vi "PH_gentec_Powermeter.destructor.vi"(0 "i ref in":refnum<vi>, 5 "error in(no error)":errorcluster) -> (19 "error out":errorcluster)   [LabVIEW 2014, in "PH_gentec_Powermeter.lvlib"]
doc: "This is the destructor of a class.\n\nLicense Agreement for this software:\n\nCopyright (C)\nGesellschaft für Schwerionenforschung, GSI\nPlanckstr. 1\n64291 Darmstadt\nGermany\n\nContact: D.Beck@gsi.de \n\nThis program is free software; you can redistribute it and/or modify it under the terms of the \nGNU General Public License as published by the Free Software Foundation; either version 2 of \nthe license, or (at your option) any later version.\n\nThis program is distributed in the hope that it will be useful, but WITHOUT ANY WARRANTY; \nwithout even the implied warranty of MERCHANTABILITY or FITNESS FOR A PARTICULAR PURPOSE. See the GNU General License for more details (http://www.gnu.org).\n\nGesellschaft für Schwerionenforschung, GSI\nPlanckstr. 1, 64291 Darmstadt, Germany\nFor all questions and ideas contact: M.Richter@gsi.de, H.Brand@gsi.de or D.Beck@gsi.de.\nLast update: 16-JUN-2004"
uses:
  PH_gentec_Powermeter.lvlib
  PH_Powermeter_BaseClass/PH_Powermeter_BaseClass.State.ctl
  PH_Powermeter_BaseClass/PH_Powermeter_BaseClass.lvlib
  non_GPL/instr.lib/gentec-SOLO-PE/gentec-SOLO-PE - Driver.lvlib
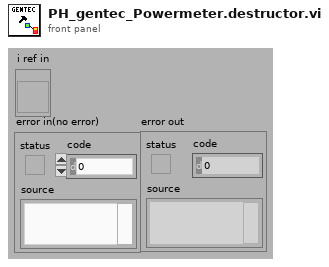
[diagram p1: front panel]
types:
  T1 = typedef "PH_Powermeter_BaseClass.lvlib/PH_Powermeter_BaseClass.State.ctl" = enum32{"off", "operating", "opened", "checked", "connected", "Sets to change", "running"}
  T2 = typedef "PH_Powermeter_BaseClass.lvlib/PH_Powermeter_BaseClass.i attribute.ctl" = cluster{"GUI References":T3, "Connection":T4, "Head Attributes":T5, "VISA resource":refnum<visa-resource-name>, "Energy":T6, "Service ID Energy":i32, "Wanted Settings":T7, "Current Settings":T7}
  T3 = typedef "PH_Powermeter_BaseClass.lvlib/PH_Powermeter_BaseClass.GUI Refs.ctl" = cluster{"Head Attributes":refnum<vi>, "Energy":refnum<vi>, "Connection":refnum<vi>, "VISA Resource":refnum<vi>, "Energy evolution":refnum<vi>, "Scaling Factor":refnum<vi>, "Range":refnum<vi>, "Wavelength":refnum<vi>, "Trigger Level":refnum<vi>, "Wanted Settings":refnum<vi>, "Current Settings":refnum<vi>}
  T4 = typedef "PH_Powermeter_BaseClass.lvlib/PH_Powermeter_BaseClass.Connection.ctl" = cluster{"failed checks":i8, "Timeout":bool, "Data read":string, "Failure":bool, "Error":bool, "State":T1}
  T5 = typedef "PH_Powermeter_BaseClass.lvlib/PH_Powermeter_BaseClass.Head Attributes.ctl" = cluster{"Instrument Type":string, "Head Version":string, "Head Name":string, "Serial Number":string, "Firmware":string, "Sensor Type":string, "MinimumRange":u32, "Maximum Range":u32, "Min Wavelength":i32, "Max Wavelength":i32}
  T6 = typedef "PH_Powermeter_BaseClass.lvlib/PH_Powermeter_BaseClass.Energy.ctl" = cluster{"current Value":dbl, "unscaled":dbl, "Scaling Factor":dbl}
  T7 = typedef "PH_Powermeter_BaseClass.lvlib/PH_gentec_BaseClass.Head Settings.ctl" = cluster{"Trigger Level":dbl, "Wavelength":u32, "Range":u32}
  T8 = enum16{"SetAttribute", "GetAttribute", "CreateAttribute", "DestroyAttribute", "DestroyAllAtributes"}
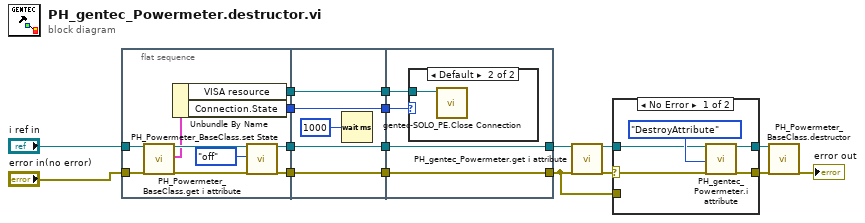
[diagram p0: block diagram]
diagram:
  n1 = flat-sequence {
    tunnel: "error in(no error)" -> [w24]
    tunnel: "i ref in" -> [w23]
    tunnel: [w26] -> w12
    tunnel: [w27] -> w11
    tunnel: [w19] -> w10
    tunnel: [w18] -> w9
    tunnel: w12 -> [w32]
    tunnel: w11 -> [w31]
    tunnel: [w32] -> w8
    tunnel: [w31] -> w7
    tunnel: w10 -> [w29]
    tunnel: [w29] -> w6
    tunnel: [w28] -> w5
    tunnel: w9 -> [w28]
    tunnel: [w34] -> w3
    tunnel: [w33] -> w2
    tunnel: w8 -> [w33]
    tunnel: w7 -> [w34]
    tunnel: w6 -> [w36]
    tunnel: w5 -> [w35]
    frame #0 {
      n2 = call "PH_Powermeter_BaseClass.get i attribute.vi"("i ref in"=w23, "error in (no error)"=w24) -> ("i ref out"=w21:refnum<vi>, "i attribute"=w20:T2, "error out"=w22:errorcluster)  [unwired: 15 in]
      n3 = Unbundle By Name(w20) -> ("VISA resource"=w19:refnum<visa-resource-name>, "Connection.State"=w18:T1)
      n4 = call "PH_Powermeter_BaseClass.set State.vi"("VI in"=w21, "State"=PH_Powermeter_BaseClass.State."off", "error in (no error)"=w22) -> ("VI out"=w27:refnum<vi>, "error out"=w26:errorcluster)  [unwired: 15 in]
    }
    frame #1 {
      n5 = Wait (ms)(milliseconds to wait=u32 1000) -> ()  [unwired: 1 out]
    }
    frame #2 {
      n6 = case shown="Default" w35 {
        tunnel: w36 -> [_ w37]
        frame "off", "operating" {
        }
        frame Default {
          n7 = call "gentec-SOLO_PE.Close Connection.vi"("VISA resource name in"=w37) -> ()  [unwired: 6 in, 1 out]
        }
      }
    }
  }
  n8 = call "PH_gentec_Powermeter.get i attribute.vi"("i ref in"=w3, "error in (no error)"=w2) -> ("i ref out"=w16:refnum<vi>, "error out"=w17:errorcluster)  [unwired: 15 in, 1 out]
  n9 = case shown="No Error" w17 {
    selector: w17 -> [w39 _]
    tunnel: [w40 w43] -> w14
    tunnel: w16 -> [w38 w44]
    tunnel: [w41 w44] -> w15
    tunnel: w2 -> [_ w43]
    frame No Error {
      n10 = call "PH_gentec_Powermeter.i attribute.vi"("VI Refnum"=w38, "Action"=T8."DestroyAttribute", "error in (no error)"=w39) -> ("VI Refnum out"=w41:refnum<vi>, "error out"=w40:errorcluster)  [unwired: 14 in, 1 out]
    }
    frame Error {
    }
  }
  n11 = call "PH_Powermeter_BaseClass.destructor.vi"("i ref in"=w15, "error in(no error)"=w14) -> ("error out"=→"error out":errorcluster)  [unwired: 17 in]
